vi "Demo_TransformImage.vi"() -> ()   [LabVIEW 2024]
doc: "Apply a transformation (rotate, skew, scale, etc) to a LV image using QuickTime\n\n© Ch. Salzmann, 1994-2003"
uses:
  <userlib>/ImageProcessing/QTLIB_2595_LV86/QT_Private.ctl
  <userlib>/ImageProcessing/QTLIB_2595_LV86/QT_Effect.ctl
panel:
  in  "Anti-aliasing (QT 6)":bool
  in  "stop":bool
  in  "Y skew":dbl format="%.2f"
  in  "X skew":dbl format="%.2f"
  in  "Y scale":dbl=1.0 format="%.2f"
  in  "X scale":dbl=1.0 format="%.2f"
  in  "Rotation angle":dbl=45.0 format="%.2f"
  out "Transformed image":picture caption="new picture"
  out "Image Source":picture
  out "error out":errorcluster
  # "Apply a transformation to a LV image\nusing QuickTime\n© Ch. Salzmann, 1994-2008"
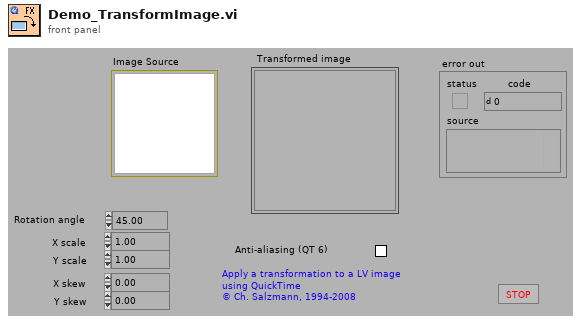
[diagram p1: front panel]
types:
  T1 = typedef "QT_Private.ctl" = cluster{"reserved 1":i32, "reserved 2":i32, "reserved 3":i32, "reserved 4":i32}
  T2 = typedef "QT_Effect.ctl" = cluster{"Reserved":i32, "Matrix":dbl[]}
  T3 = typedef "QT_Image.ctl" = cluster{"Width":i32, "Height":i32, "Depth":i32, "data":u8[], "Compressed data":u8[], "Color table":u32[], "Duration":i32, "Options":i32, "Timestamp":i32, "ID":i32, "Reserved":i32, "Dialogs":u32}
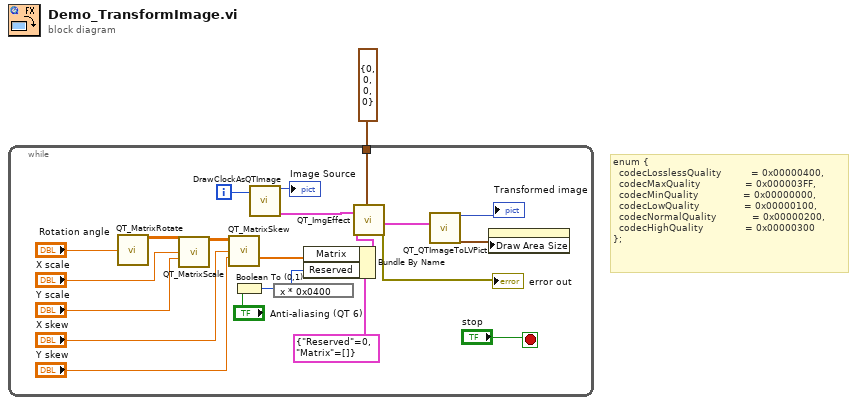
[diagram p0: block diagram]
diagram:
  # "enum {\n  codecLosslessQuality          = 0x00000400,\n  codecMaxQuality               = 0x000003FF,\n  codecMinQuality               = 0x00000000,\n  codecLowQuality               = 0x00000100,\n  codecNormalQuality            = 0x00000200,\n  codecHighQuality              = 0x00000300\n};"
  n1 = while {
    tunnel: T1 {"reserved 1"=0, "reserved 2"=0, "reserved 3"=0, "reserved 4"=0} ("Private") -> [w2]
    i -> [w20]
    stop <- "stop" stop-if-true
    n2 = call <userlib>:"QT_MatrixRotate.vi"("Angle [deg]"="Rotation angle") -> ("Out Matrix"=w18:dbl[][])  [unwired: 4 in, 10 out]
    n3 = call <userlib>:"QT_MatrixScale.vi"("In Matrix [3x3] (Identity)"=w18, "X scale"="X scale", "Y scale"="Y scale") -> ("Out Matrix"=w15:dbl[][])  [unwired: 1 in, 11 out]
    n4 = call <userlib>:"QT_MatrixSkew.vi"("In Matrix [3x3] (Identity)"=w15, "X skew"="X skew", "Y skew"="Y skew") -> ("Out Matrix as Vector"=w8:dbl[])  [unwired: 1 in, 11 out]
    n5 = Boolean To (0,1)(Boolean="Anti-aliasing (QT 6)") -> (0, 1=w3:i16)
    n6 = call <userlib>:"DrawClockAsQTImage.vi"("frame ID"=w20) -> ("Picture"=→"Image Source":picture, "Image Out (24 bits)"=w23:T3)  [unwired: 1 in, 16 out]
    n7 = expression code="x * 0x0400"(w3) -> (w5:i16)
    n8 = Bundle By Name(cluster=T2 {"Reserved"=0, "Matrix"=[]} ("Effect"), "Matrix"=w8, "Reserved"=w5) -> (w22:T2)
    n9 = call <userlib>:"QT_ImgEffect.vi"("Image In"=w23, "Effect"=w22, "Private"=w2) -> ("Image Out"=w13:T3, "error out"=→"error out":errorcluster)  [unwired: 2 in, 13 out]
    n10 = call <userlib>:"QT_QTImageToLVPict.vi"("Image/Movie Out"=w13) -> ("Picture color"=→"Transformed image":picture, "Pict Draw Area Size"=w11:cluster{"Width":i16, "Height":i16})  [unwired: 2 in, 15 out]
    n11 = property on="Transformed image" class="Pict"("Draw Area Size"=w11) -> ()  [unwired: 2 in, 2 out]
  }
